vi "HandleCheat.vi"(8 "error in (no error)":errorcluster, 11 "Engine in":refnum<class "Engine.lvclass">) -> (0 "error out":errorcluster, 3 "Engine out":refnum<class "Engine.lvclass">)   [LabVIEW 2019]
uses:
  CheatGlobals.vi
  Engine.lvclass
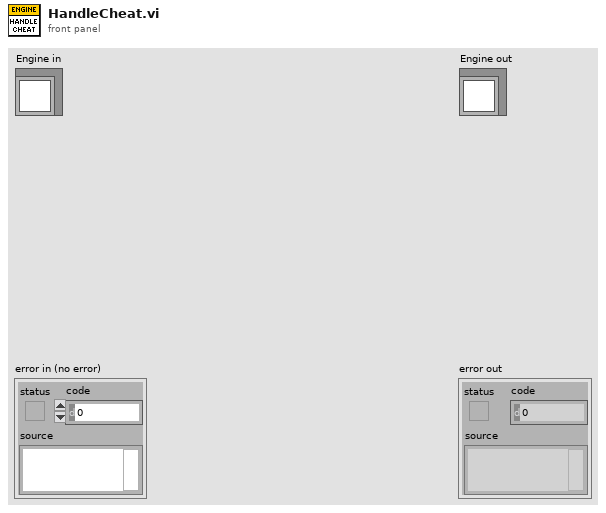
[diagram p1: front panel]
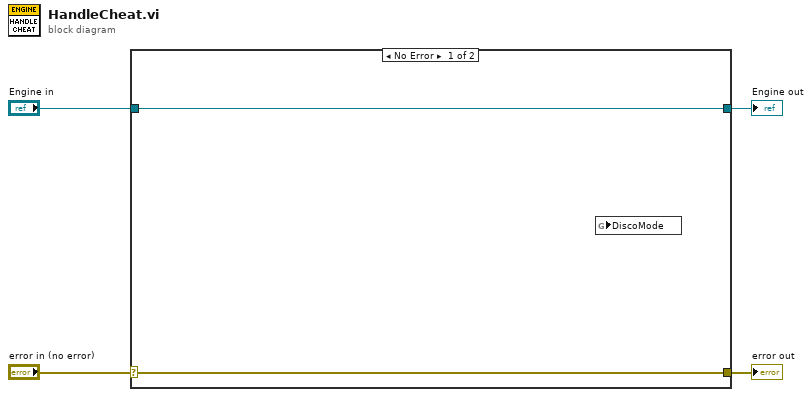
[diagram p0: block diagram]
diagram:
  n1 = case shown="No Error" "error in (no error)" {
    selector: "error in (no error)" -> [w5 w8]
    tunnel: [w5 w8] -> w3
    tunnel: [w6 w7] -> w1
    tunnel: "Engine in" -> [w6 w7]
    frame No Error {
      n2 = global read "CheatGlobals.vi" "DiscoMode"() -> ()  [unwired: 1 in]
    }
    frame Error {
    }
  }
  "error out" <- w3
  "Engine out" <- w1
